vi "FPGA IIR 24th order Core.vi"(0 "input data":fxp<+/-,20,5>, 1 "coeff_a":fxp<+/-,22,4>[](array[numeric])=[0.0, 0.0, 0.0, 0.0, 0.0, 0.0, 0.0, 0.0, 0.0, 0.0, 0.0, 0.0, 0.0, 0.0, 0.0, 0.0, 0.0, 0.0, 0.0, 0.0, 0.0, 0.0, 0.0, 0.0, 0.0, 0.0, 0.0, 0.0, 0.0, 0.0, 0.0, 0.0, 0.0, 0.0, 0.0, 0.0], 2 "coeff_b":fxp<+/-,22,4>[](array[numeric])=[1.0, 0.0, 0.0, 1.0, 0.0, 0.0, 1.0, 0.0, 0.0, 1.0, 0.0, 0.0, 1.0, 0.0, 0.0, 1.0, 0.0, 0.0, 1.0, 0.0, 0.0, 1.0, 0.0, 0.0, 1.0, 0.0, 0.0, 1.0, 0.0, 0.0, 1.0, 0.0, 0.0, 1.0, 0.0, 0.0], 9 "input valid":bool, 12 "reset":bool) -> (4 "output data":fxp<+/-,20,5> format="%.31g", 10 "output valid":bool, 14 "ready for input":bool)   [LabVIEW 2011]
doc: "----------------------\n\nThis filter is configured as follows:\n\n<b>Filter Configuration</b>\nType: Single Rate\nStructure: IIR Cascaded Second-Order Sections Form II Transposed\n\n<b>Input Data Type</b>\nType: fixed-point <±,20,5> [-1.600000E+1,1.599997E+1]:3.051758E-5\n\n<b>Output Data Type</b>\nType: fixed-point <±,20,5> [-1.600000E+1,1.599997E+1]:3.051758E-5\nRounding mode: Round-Half-Even\nOverflow mode: Wrap\n\n<b>Implementation</b>\nNumber of channels: 8\nMaximum input sampling rate per channel @ 40MHz: 138.889kHz\nGain processing: On Host\nMethod: Multiply-Accumulate\n\n<b>Execution Mode</b>\nInside single-cycle Timed Loop\nThroughput: 36 cycles/sample\n\n<b>Estimated Resources</b>\n2 22x32 multiplier"
uses:
  <vilib>/rvi/FXPMathLib/FxpMul/XNode/nifxpmath_Multiplier.xnode
  <vilib>/rvi/FXPMathLib/basic elements/FxpDiscreteDelay/XNode/nifxpmath_DiscreteDelay.xnode
  <vilib>/rvi/FXPMathLib/sim/FxpSim.dll
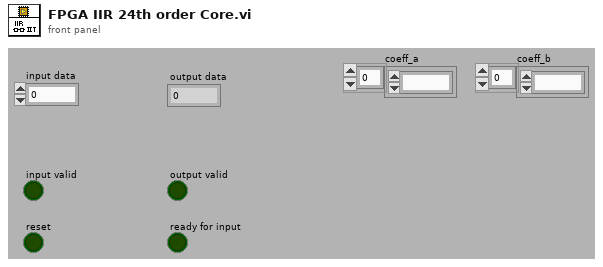
[diagram p1: front panel]
types:
  T1 = cluster{"update  v?":bool, "write s1?":bool, "init?":bool}
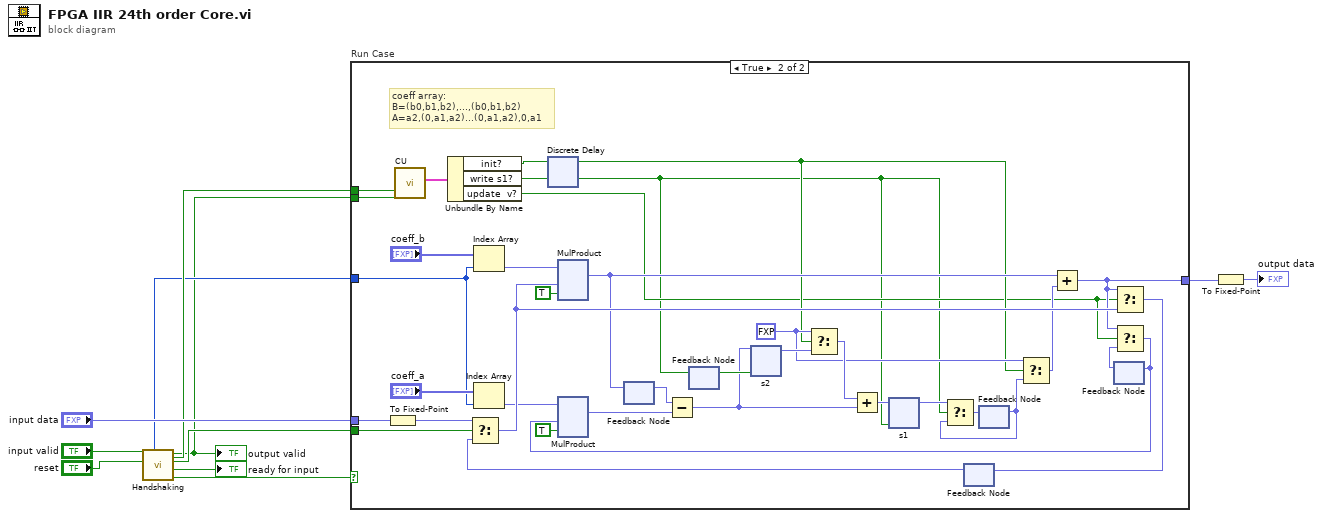
[diagram p0: block diagram]
diagram:
  n1 = call "Handshaking"("reset"="reset", "input valid"="input valid") -> ("run?"=w8:bool, "ready for input"=→"ready for input":bool, "load"=w4:bool, "output valid"=w1:bool, "reset for cu"=w7:bool, "idx"=w5:i16)  [unwired: 4 out]
  "output valid" <- w1
  n2 = case "Run Case" shown="True" w8 {
    tunnel: "input data" -> [_ w19]
    tunnel: w1 -> [_ w40]
    tunnel: w4 -> [_ w20]
    tunnel: w7 -> [_ w39]
    tunnel: w5 -> [_ w21]
    tunnel: [_ w22] -> w2
    frame False {
    }
    frame True {
      w28 = fxp<+/-,64,33> 0.0 ("kDelay")
      # "coeff array:\nB=(b0,b1,b2),...,(b0,b1,b2)\nA=a2,(0,a1,a2)...(0,a1,a2),0,a1"
      n3 = To Fixed-Point ("toMultiplicand")(number=w19) -> (fixed-point=w44:fxp<+/-,64,33>)  [unwired: 1 out]
      n4 = call "CU"("output valid"=w40, "global reset"=w39) -> ("Control signal"=w27:T1)  [unwired: 9 out]
      n5 = Unbundle By Name(w27) -> ("init?"=w38:bool, "write s1?"=w14:bool, "update  v?"=w15:bool)
      n6 = Index Array(array="coeff_b", index=w21) -> (element=w43:fxp<+/-,22,4>)
      n7 = Index Array(array="coeff_a", index=w21) -> (element=w29:fxp<+/-,22,4>)
      n8 = xnode ("Discrete Delay")("D"=w38) -> ("Q"=w16:bool)
      n9 = feedback #1() -> (w33:fxp<+/-,64,37>)  [unwired: 1 out]
      n10 = feedback-in #2(w14) -> ()
      n11 = feedback #2() -> (w35:bool)  [unwired: 1 out]
      n12 = feedback #3() -> (w41:fxp<+/-,64,33>)  [unwired: 1 out]
      n13 = Select(t=w44, s=w20, f=w41) -> (s? t:f=w42:fxp<+/-,64,33>)
      n14 = xnode ("MulProduct")("x"=w43, "y"=w42, "input valid"=TRUE) -> ("x*y"=w18:fxp<+/-,64,37>)  [unwired: 1 in, 2 out]
      n15 = feedback-in #1(w18) -> ()
      n16 = feedback #4() -> (w30:fxp<+/-,64,33>)  [unwired: 1 out]
      n17 = Select(t=w28, s=w16, f=w30) -> (s? t:f=w17:fxp<+/-,64,33>)
      n18 = Add ("AddSum")(x=w18, y=w17) -> (x+y=w22:fxp<+/-,64,33>)
      n19 = feedback #5() -> (w34:fxp<+/-,64,33>)  [unwired: 1 out]
      n20 = Select(t=w22, s=w15, f=w42) -> (s? t:f=w24:fxp<+/-,64,33>)
      n21 = feedback-in #3(w24) -> ()
      n22 = Select(t=w22, s=w15, f=w34) -> (s? t:f=w23:fxp<+/-,64,33>)
      n23 = xnode ("MulProduct")("x"=w29, "y"=w23, "input valid"=TRUE) -> ("x*y"=w45:fxp<+/-,64,37>)  [unwired: 1 in, 2 out]
      n24 = Subtract ("SubSum")(x=w33, y=w45) -> (x-y=w25:fxp<+/-,64,33>)
      n25 = xnode ("s2")("D"=w25, "enable"=w35) -> ("Q"=w36:fxp<+/-,64,33>)
      n26 = Select(t=w28, s=w16, f=w36) -> (s? t:f=w37:fxp<+/-,64,33>)
      n27 = Add ("AddSum")(x=w37, y=w25) -> (x+y=w26:fxp<+/-,64,33>)
      n28 = xnode ("s1")("D"=w26, "enable"=w14) -> ("Q"=w32:fxp<+/-,64,33>)
      n29 = Select(t=w32, s=w14, f=w30) -> (s? t:f=w31:fxp<+/-,64,33>)
      n30 = feedback-in #4(w31) -> ()
      n31 = feedback-in #5(w23) -> ()
    }
  }
  n32 = To Fixed-Point ("toOutput")(number=w2) -> (fixed-point=→"output data":fxp<+/-,20,5>)  [unwired: 1 out]
